vi "Update Flow.vi"(8 "error in":errorcluster, 9 "Status":map{string, bool}(c390), 10 "Flow":sgl, 11 "DeepU Results in":refnum<class "DeepU Results.lvclass">) -> (0 "error out":errorcluster, 3 "DeepU Results out":refnum<class "DeepU Results.lvclass">)   [LabVIEW 2019, in "Results.lvlib" / "DeepU Results.lvclass"]
uses:
  DeepU Results.lvclass
  DeepU Results.lvclass/DeepU Results.ctl
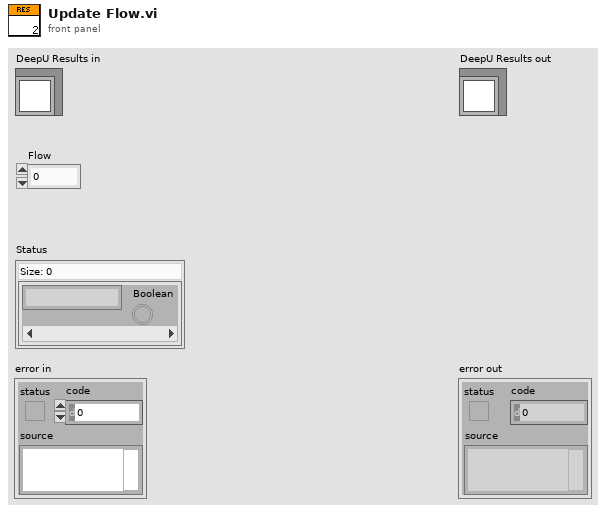
[diagram p1: front panel]
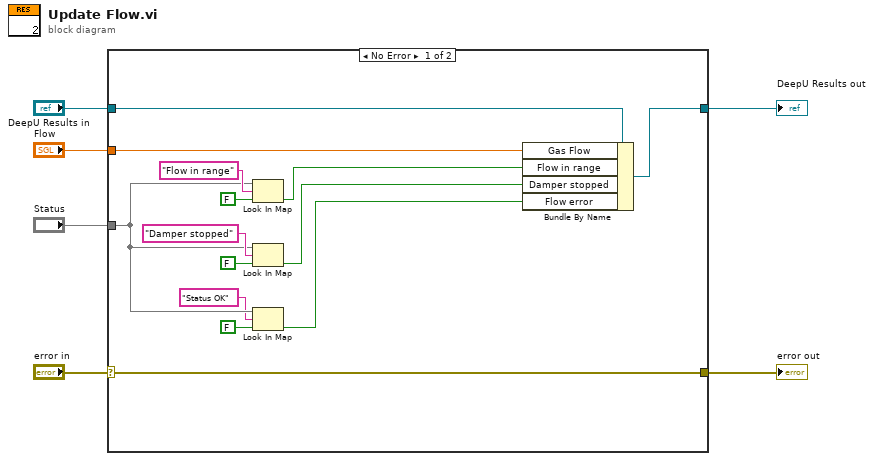
[diagram p0: block diagram]
diagram:
  n1 = case shown="No Error" "error in" {
    selector: "error in" -> [w19 w22]
    tunnel: [w19 w22] -> w5
    tunnel: [w18 w21] -> w3
    tunnel: "DeepU Results in" -> [w20 w21]
    tunnel: "Flow" -> [w17 _]
    tunnel: "Status" -> [w12 _]
    frame No Error {
      n2 = Look In Map(map=w12, key="Flow in range", default value=FALSE) -> (value=w15:bool)  [unwired: 1 out]
      n3 = Look In Map(map=w12, key="Damper stopped", default value=FALSE) -> (value=w13:bool)  [unwired: 1 out]
      n4 = Look In Map(map=w12, key="Status OK", default value=FALSE) -> (value=w10:bool)  [unwired: 1 out]
      n5 = Bundle By Name(cluster=w20, "Gas Flow"=w17, "Flow in range"=w15, "Damper stopped"=w13, "Flow error"=w10) -> (w18:refnum<class "DeepU Results.lvclass">)
    }
    frame Error {
    }
  }
  "error out" <- w5
  "DeepU Results out" <- w3
